vi "NI VeriStand - Search for All Items by Property.vi"(8 "error in":errorcluster, 9 "Property Value":variant, 10 "Property Name":string, 11 "Section Ref in":T1 format="%.0x") -> (0 "error out":errorcluster, 2 "Item Refs":T1[](array[typedef]) format="%.0x", 3 "Section Ref out":T1 format="%.0x", 4 "Found":bool)   [LabVIEW 2020, in "Custom Device Utility Library.lvlib"]
doc: "Searches a custom device section for the item(s) you specify. You can search for one or multiple items by name, GUID, or property name and value. You must manually select the polymorphic instance to use."
uses:
  <vilib>/NI VeriStand/Custom Device Tools/Custom Device Utility Library/Custom Device Utility Library.lvlib
  <vilib>/NI VeriStand/Custom Device API/Custom Device Item Ref.ctl
  <vilib>/NI VeriStand/Custom Device API/Get Item Property (Variant).vi
  <vilib>/NI VeriStand/Custom Device API/Custom Device API.lvlib
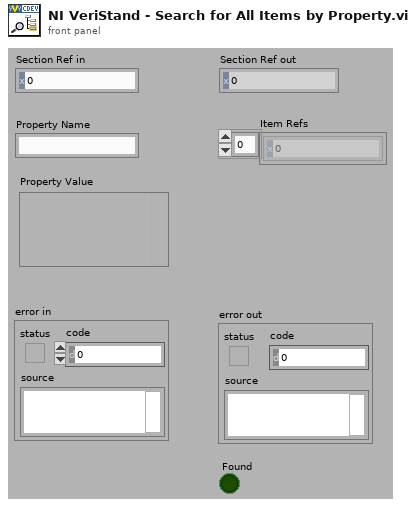
[diagram p1: front panel]
types:
  T1 = typedef "Custom Device API.lvlib/Custom Device Item Ref.ctl" = u64
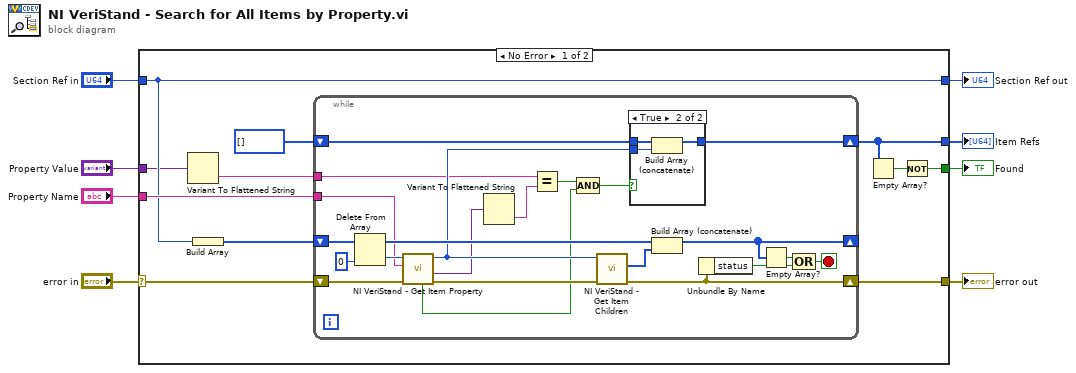
[diagram p0: block diagram]
diagram:
  n1 = case shown="No Error" "error in" {
    selector: "error in" -> [w12 w47]
    tunnel: "Section Ref in" -> [w11 w46]
    tunnel: "Property Name" -> [w18 _]
    tunnel: [w17 w47] -> w6
    tunnel: [w15 _] -> w5
    tunnel: [w13 _] -> w4
    tunnel: [w11 w46] -> w2
    tunnel: "Property Value" -> [w10 _]
    frame No Error {
      n2 = Variant To Flattened String(Variant=w10) -> (data string=w9:string)  [unwired: 1 out]
      n3 = Build Array(w11) -> (w19:T1[])
      n4 = while {
        shift-right: [w41] -> w17
        shift-left: w12 -> [w39]
        shift-right: [w33] -> _
        shift-left: w19 -> [w38]
        tunnel: w18 -> [w26]
        shift-right: [w28] -> w15
        shift-left: T1[] [] ("appended array") -> [w29]
        tunnel: w9 -> [w25]
        stop <- w30 stop-if-true
        n5 = Delete From Array(array=w38, index=0) -> (deleted portion=w36:T1, array with subset deleted=w35:T1[])  [unwired: 1 in]
        n6 = call-poly <vilib>:"NI VeriStand - Get Item Property.vi"("error in (no error)"=w39, "Property Name"=w26, "Item Ref in"=w36) -> ("error out"=w40:errorcluster, "Value"=w21:variant, "Item Ref out"=w27:T1, "Found?"=w23:bool)  [unwired: 1 in, 4 out]
        n7 = Variant To Flattened String(Variant=w21) -> (data string=w20:string)  [unwired: 1 out]
        n8 = Equal?(x=w25, y=w20) -> (x = y?=w24:bool)
        n9 = Compound Arithmetic op=AND(w24, w23) -> (w22:bool)
        n10 = call <vilib>:"NI VeriStand - Get Item Children.vi"("error in (no error)"=w40, "Item Ref in"=w27) -> ("error out"=w41:errorcluster, "Child Refs"=w34:T1[])  [unwired: 8 out]
        n11 = case shown="True" w22 {
          tunnel: w29 -> [w42 w45]
          tunnel: [w42 w44] -> w28
          tunnel: w27 -> [_ w43]
          frame False {
          }
          frame True {
            n12 = Build Array (concatenate)(w45, w43) -> (w44:T1[])
          }
        }
        n13 = Build Array (concatenate)(w35, w34) -> (w33:T1[])
        n14 = Unbundle By Name(w41) -> ("status"=w32:bool)
        n15 = Empty Array?(array=w33) -> (empty?=w31:bool)
        n16 = Compound Arithmetic op=OR(w31, w32) -> (w30:bool)
      }
      n17 = Empty Array?(array=w15) -> (empty?=w14:bool)
      n18 = Not(x=w14) -> (.not. x?=w13:bool)
    }
    frame Error {
    }
  }
  "Found" <- w4
  "error out" <- w6
  "Section Ref out" <- w2
  "Item Refs" <- w5
